vi "Menu-Stop Log.vi"(8 "error in":errorcluster, 11 "Menu in":refnum<k9>) -> ()   [LabVIEW 2016, in "CML UI.lvlib"]
uses:
  CML UI.lvlib
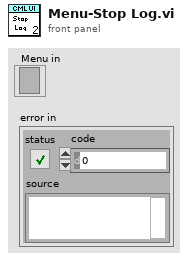
[diagram p1: front panel]
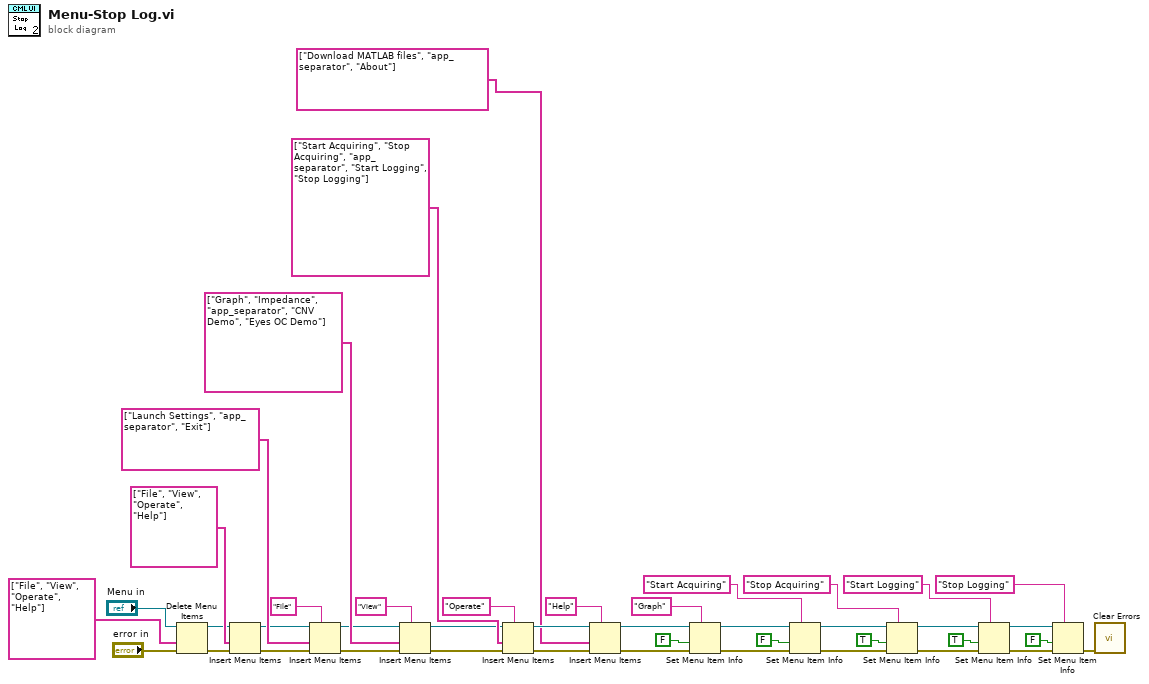
[diagram p0: block diagram]
diagram:
  n1 = Delete Menu Items(6:"error in", 7:string[] ["File", "View", "Operate", "Help"] ("L10n_item tags 1"), 9:"Menu in") -> (0:w19:errorcluster, 3:w20:refnum<k9>)  [unwired: 1 in]
  n2 = Insert Menu Items(6:w19, 7:string[] ["File", "View", "Operate", "Help"] ("L10n_item tags 1"), 9:w20) -> (0:w32:errorcluster, 3:w30:refnum<k9>)  [unwired: 3 in, 1 out]
  n3 = Insert Menu Items(5:"File" ("L10n_menu tag"), 6:w32, 7:string[] ["Launch Settings", "app_separator", "Exit"] ("L10n_item tags 2"), 9:w30) -> (0:w37:errorcluster, 3:w36:refnum<k9>)  [unwired: 2 in, 1 out]
  n4 = Insert Menu Items(5:"View" ("L10n_menu tag"), 6:w37, 7:string[] ["Graph", "Impedance", "app_separator", "CNV Demo", "Eyes OC Demo"] ("L10n_item tags 2"), 9:w36) -> (0:w41:errorcluster, 3:w40:refnum<k9>)  [unwired: 2 in, 1 out]
  n5 = Insert Menu Items(5:"Operate" ("L10n_menu tag"), 6:w41, 7:string[] ["Start Acquiring", "Stop Acquiring", "app_separator", "Start Logging", "Stop Logging"] ("L10n_item tags 2"), 9:w40) -> (0:w27:errorcluster, 3:w28:refnum<k9>)  [unwired: 2 in, 1 out]
  n6 = Insert Menu Items(5:"Help" ("L10n_menu tag"), 6:w27, 7:string[] ["Download MATLAB files", "app_separator", "About"] ("L10n_item tags 2"), 9:w28) -> (0:w24:errorcluster, 3:w26:refnum<k9>)  [unwired: 2 in, 1 out]
  n7 = Set Menu Item Info(7:"Graph" ("item tag"), 8:w24, 9:FALSE ("enabled"), 11:w26) -> (0:w6:errorcluster, 3:w7:refnum<k9>)  [unwired: 3 in]
  n8 = Set Menu Item Info(7:"Start Acquiring" ("item tag"), 8:w6, 9:FALSE ("enabled"), 11:w7) -> (0:w4:errorcluster, 3:w5:refnum<k9>)  [unwired: 3 in]
  n9 = Set Menu Item Info(7:"Stop Acquiring" ("item tag"), 8:w4, 9:TRUE ("enabled"), 11:w5) -> (0:w13:errorcluster, 3:w14:refnum<k9>)  [unwired: 3 in]
  n10 = Set Menu Item Info(7:"Start Logging" ("item tag"), 8:w13, 9:TRUE ("enabled"), 11:w14) -> (0:w11:errorcluster, 3:w12:refnum<k9>)  [unwired: 3 in]
  n11 = Set Menu Item Info(7:"Stop Logging" ("item tag"), 8:w11, 9:FALSE ("enabled"), 11:w12) -> (0:w10:errorcluster)  [unwired: 3 in, 1 out]
  n12 = call <vilib>:"Clear Errors.vi"("error in (no error)"=w10) -> ()  [unwired: 5 in, 2 out]
